vi "asdfa.vi"() -> ()   [LabVIEW 2009]
panel:
  out "Boolean array":bool[](array[boolean])
  in  "Numeric":u8
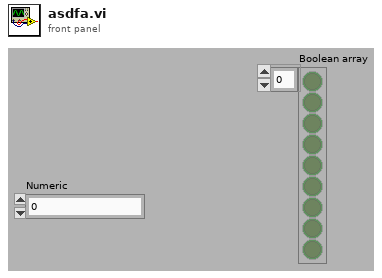
[diagram p1: front panel]
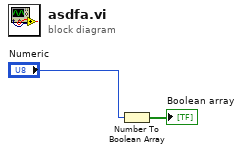
[diagram p0: block diagram]
diagram:
  n1 = Number To Boolean Array(number="Numeric") -> (Boolean array=→"Boolean array":bool[])
